vi "Periodic Tasks.vi"(8 "error in (no error)":errorcluster) -> ()   [LabVIEW 2011]
doc: "This VI runs in parallel to other tasks. It can contain as many user-defined periodic loops as you need. These can carry out PID or other sorts of timed response."
uses:
  <vilib>/addons/Kinect/SkeletonVertexTrackState.ctl
  <vilib>/Rock Robotics/SystemInterfaces/Utilities/FPGA_UtilitiesLED State.ctl
  <vilib>/Rock Robotics/SystemInterfaces/Utilities/FPGA_UtilitiesLED Source.ctl
  <vilib>/Rock Robotics/WPI/Solenoid/WPI_SolenoidValue.ctl
  <vilib>/Rock Robotics/WPI/CAN/Jaguar/SubVIs/WPI_CANJaguar_StatusSelect.ctl
  <vilib>/Rock Robotics/WPI/Compressor/WPI_CompressorGetSetRefNum.vi
  Robot Global Data.vi
  <vilib>/Rock Robotics/WPI/Solenoid/Deprecated/WPI_SolenoidGetBool.vi
  <vilib>/Rock Robotics/WPI/Solenoid/WPI_SolenoidSetEnum.vi
panel:
  out "Skeleton Tracking State":T1[](array[typedef])
  out "index":i32
  out "Target Locked":bool
  out "is not locked":bool
  out "is locked":bool
  out "Actual RPM":dbl
  out "Calculated RPM":dbl
  out "small error":bool
  out "poutput":dbl
  out "Distance from dash":dbl
  out "lr-v-out":dbl
  in  "Distance":dbl
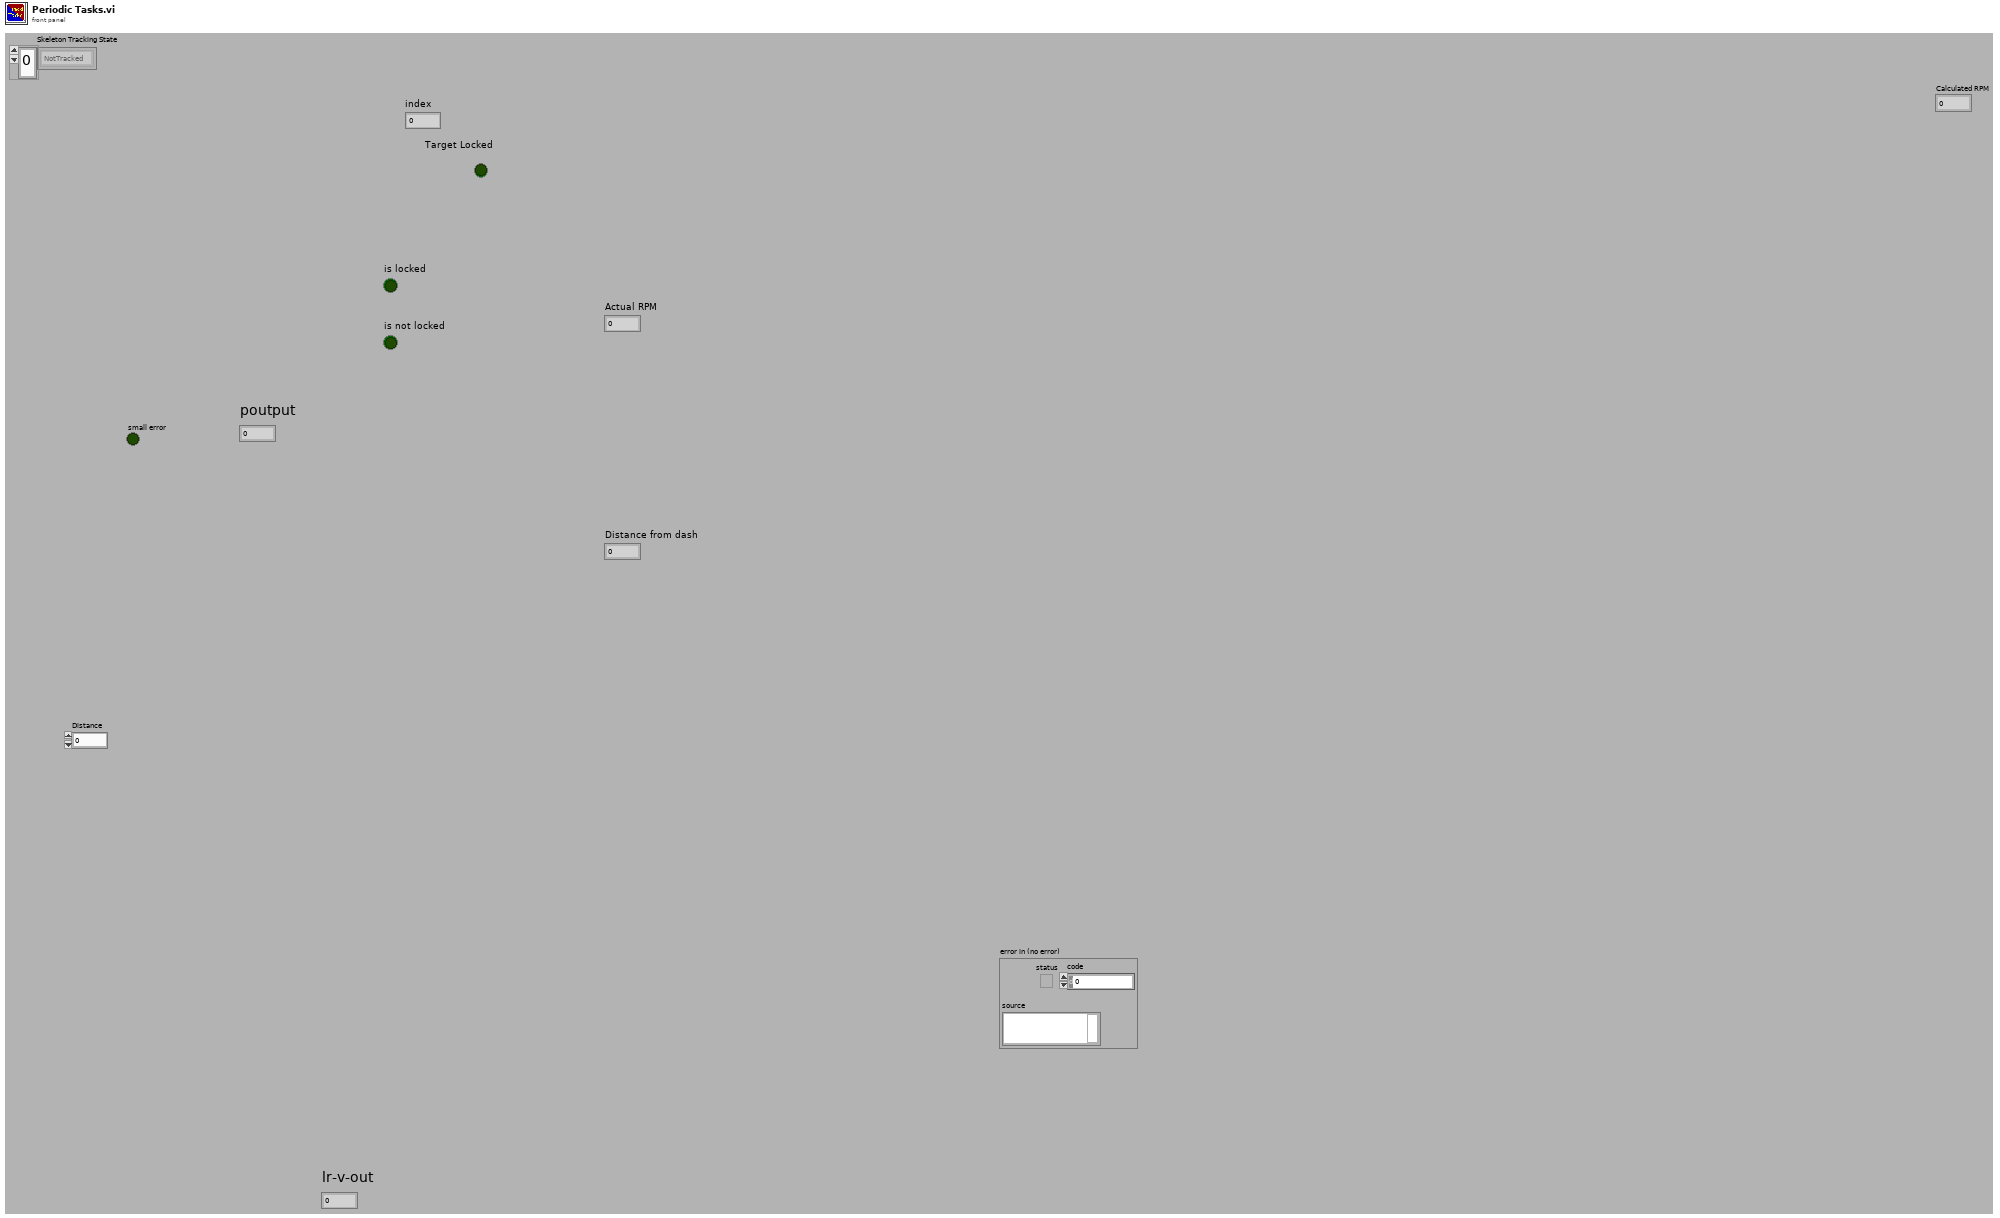
[diagram p1: front panel]
types:
  T1 = typedef "SkeletonVertexTrackState.ctl" = enum32{"NotTracked", "Inferred", "Tracked"}
  T2 = typedef "FPGA_UtilitiesLED State.ctl" = enum16{"Off", "On", "Toggle"}
  T3 = typedef "FPGA_UtilitiesLED Source.ctl" = enum16{"User LED", "FPGA LED"}
  T4 = typedef "WPI_CompressorDevRef.ctl" = cluster{"DevStatus":errorcluster, "DigitalInputDevRef":T5, "RelayDevRef":T8}
  T5 = typedef "WPI_DigitalInputDevRef.ctl" = cluster{"DevStatus":errorcluster, "DIO Channel":T6, "Digital Module":T7}
  T6 = typedef "FPGA_DIOChannel.ctl" = enum8{"DIO 1", "DIO 2", "DIO 3", "DIO 4", "DIO 5", "DIO 6", "DIO 7", "DIO 8", "DIO 9", "DIO 10", "DIO 11", "DIO 12", "DIO 13", "DIO 14", "Invalid"}
  T7 = typedef "FPGA_TypedefDigitalModule.ctl" = enum16{"Digital Module 1", "Digital Module 2"}
  T8 = typedef "WPI_RelayDevRef.ctl" = cluster{"DevStatus":errorcluster, "Relay Channel":T9, "Digital Module":T7, "Relay Direction":T10}
  T9 = typedef "FPGA_DIORelayChannel.ctl" = enum8{"Relay 1", "Relay 2", "Relay 3", "Relay 4", "Relay 5", "Relay 6", "Relay 7", "Relay 8", "Invalid"}
  T10 = typedef "WPI_RelayDirection.ctl" = enum16{"Both directions", "Forward only", "Reverse only"}
  T11 = typedef "WPI_SolenoidValue.ctl" = enum16{"Off", "On", "Forward", "Reverse"}
  T12 = typedef "WPI_JoystickDevRef.ctl" = cluster{"Device":T13}
  T13 = typedef "WPI_JoystickDeviceEnum.ctl" = enum16{"USB 1", "USB 2", "USB 3", "USB 4", "Kinect 1", "Kinect 2"}
  T14 = cluster{"axis 1 (x)":dbl, "axis 2 (y)":dbl, "axis 3 (throttle)":dbl, "axis 4":dbl, "axis 5":dbl, "axis 6":dbl}
  T15 = cluster{"RightAxis":dbl, "LeftAxis":dbl, "RightHead":bool, "Left Head":bool, "Left Leg Out":bool, "Left Leg Forward":bool, "Left Leg Back":bool, "Right Leg Out":bool, "Right Leg Forward":bool, "Right Leg Back":bool}
  T16 = typedef "WPI_SolenoidDevRef.ctl" = cluster{"DevStatus":errorcluster, "Solenoid Module":T17, "Forward Solenoid Channel":T18, "Reverse Solenoid Channel":T18}
  T17 = typedef "FPGA_TypedefSolenoidModule.ctl" = enum16{"Solenoid Module 1", "Solenoid Module 2"}
  T18 = typedef "WPI_SolenoidChannel.ctl" = enum8{"Solenoid 1", "Solenoid 2", "Solenoid 3", "Solenoid 4", "Solenoid 5", "Solenoid 6", "Solenoid 7", "Solenoid 8", "Invalid"}
  T19 = typedef "WPI_JoystickButtonState.ctl" = cluster{"Button 1":bool, "Button 2":bool, "Button 3":bool, "Button 4":bool, "Button 5":bool, "Button 6":bool, "Button 7":bool, "Button 8":bool, "Button 9":bool, "Button 10":bool, "Button 11":bool, "Button 12":bool}
  T20 = typedef "WPI_CANJaguar_StatusSelect.ctl" = enum16{"Output Percent VBus", "Output Voltage", "Bus Voltage", "Current", "Temperature", "Position", "Speed", "Limit Switches", "Faults", "Fault Counters", "Power Cycle"}
  T21 = typedef "WPI_MotorControlDeviceRef.ctl" = cluster{"DeviceStatus":errorcluster, "Type":enum16{"PWM", "CAN"}, "PWM":cluster{"Digital Module":T7, "PWM Channel":T22, "DeadBand":T23}, "CAN":cluster{"Device Number":u8, "Control Mode":T24, "Semaphore":T25, "Max Vout":dbl}, "Invert":bool, "TransformRef":T26, "InvTransformRef":T26}
  T22 = typedef "FPGA_DIOPWMChannel.ctl" = enum8{"PWM 1", "PWM 2", "PWM 3", "PWM 4", "PWM 5", "PWM 6", "PWM 7", "PWM 8", "PWM 9", "PWM 10", "Invalid"}
  T23 = typedef "WPI_PWMDeadband.ctl" = cluster{"Name":string, "maxPositivePwm":i32, "minPositivePwm":i32, "centerPwm":i32, "maxNegativePwm":i32, "minNegativePwm":i32, "angularRange":u16}
  T24 = typedef "WPI_CANJaguar_ControlMode.ctl" = enum8{"Percent VBus", "Current", "Speed", "Position", "Voltage"}
  T25 = typedef "Semaphore RefNum" = refnum<k1>
  T26 = typedef "WPI_PWMTransform_ConPane.ctl" = refnum<vi>
  T27 = typedef "WPI_CANJaguar_Status.ctl" = cluster{"Output Percent VBus":dbl, "Output Voltage":dbl, "Bus Voltage":dbl, "Current":dbl, "Temperature":dbl, "Position":dbl, "Speed":dbl, "Limits":cluster{"Forward Limit":bool, "Reverse Limit":bool, "Forward Soft Limit":bool, "Reverse Soft Limit":bool, "Sticky Forward Limit":bool, "Sticky Reverse Limit":bool, "Sticky Forward Soft Limit":bool, "Sticky Reverse Soft Limit":bool}, "Faults":cluster{"Current Fault":bool, "Temperature Fault":bool, "Bus Voltage Fault":bool, "Gate Driver Fault":bool, "Comm Fault":bool}, "Fault Counters":cluster{"Current Faults":u8, "Temperature Faults":u8, "Bus Voltage Faults":u8, "Gate Driver Faults":u8, "Comm Faults":u8, "CAN Status":u8, "CAN RX Errors":u8, "CAN TX Errors":u8}, "Power Cycle":bool}
  T28 = typedef "WPI_DigitalOutputDevRef.ctl" = cluster{"Digital Module":T7, "DIO Channel":T6, "DevStatus":errorcluster}
  T29 = cluster{"Selected Distance":dbl, "Calculated RPM":dbl, "Actual RPM":dbl, "Target Locked":bool}
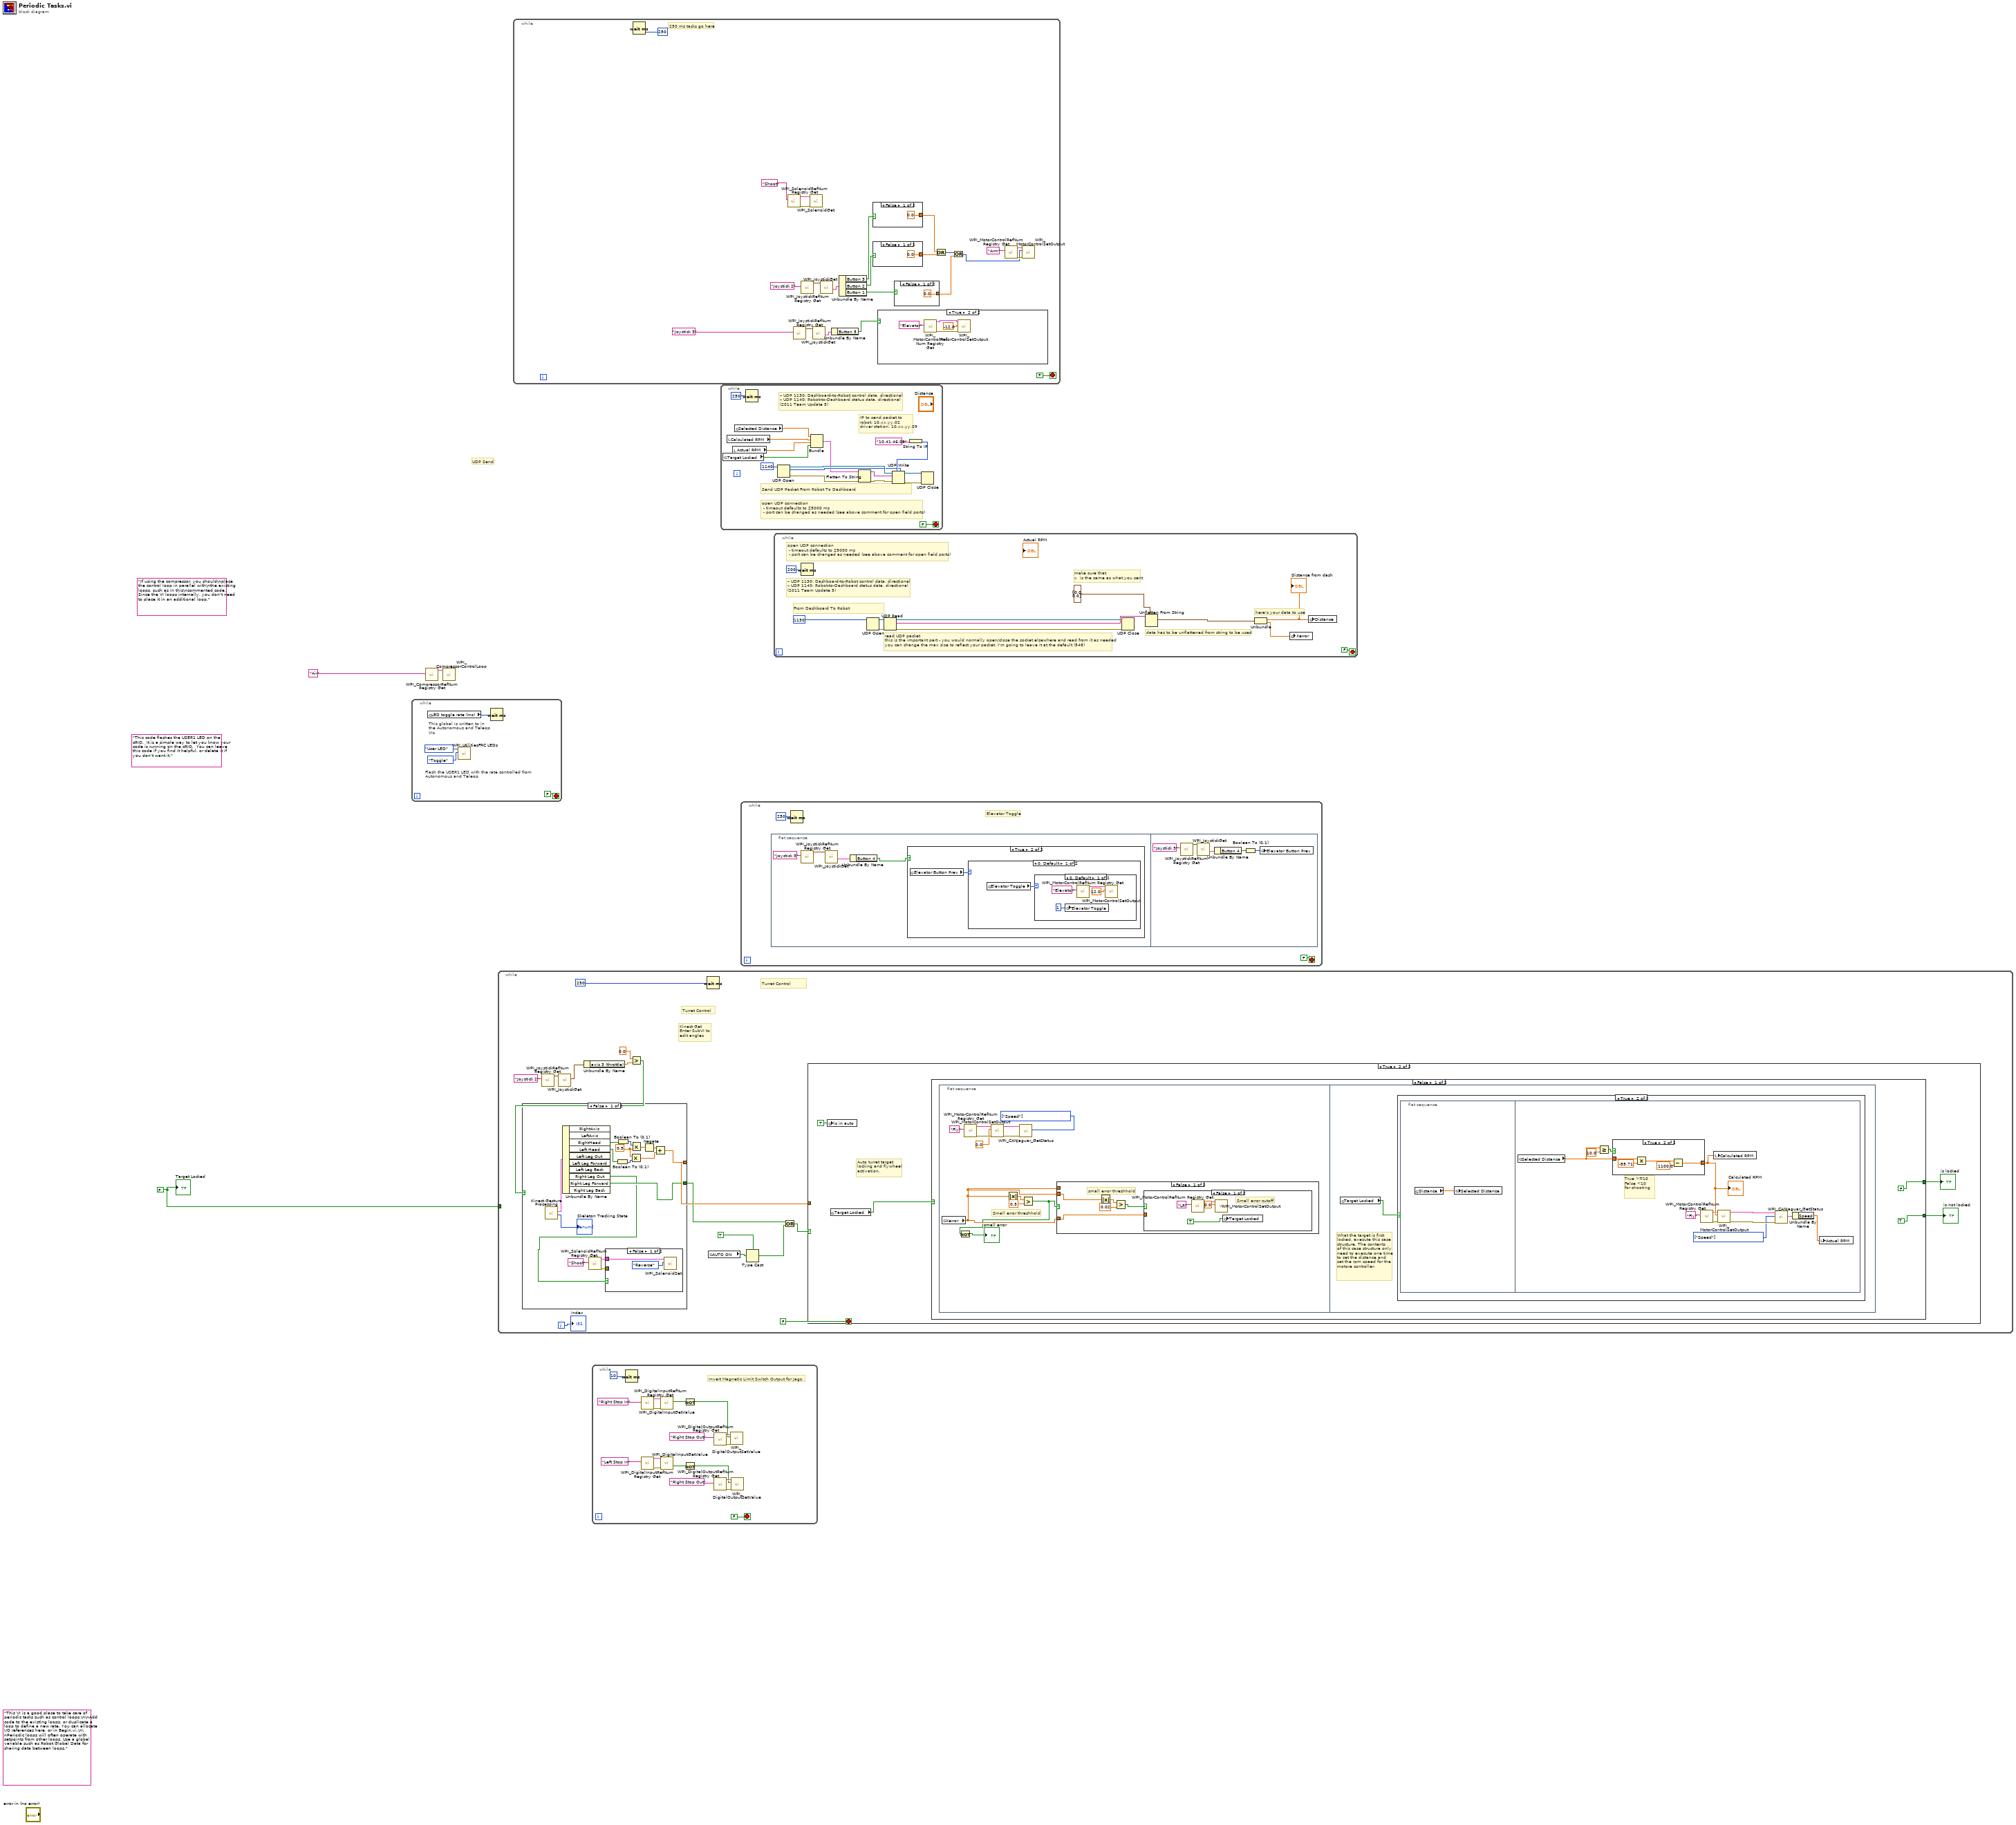
[diagram p0: block diagram]
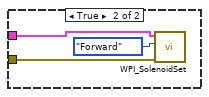
[diagram p2: hidden frame]
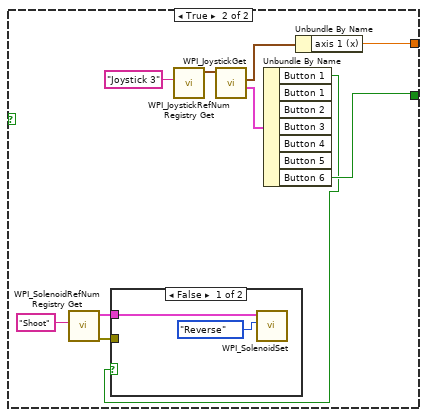
[diagram p3: hidden frame]
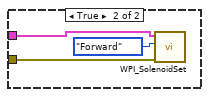
[diagram p4: hidden frame]
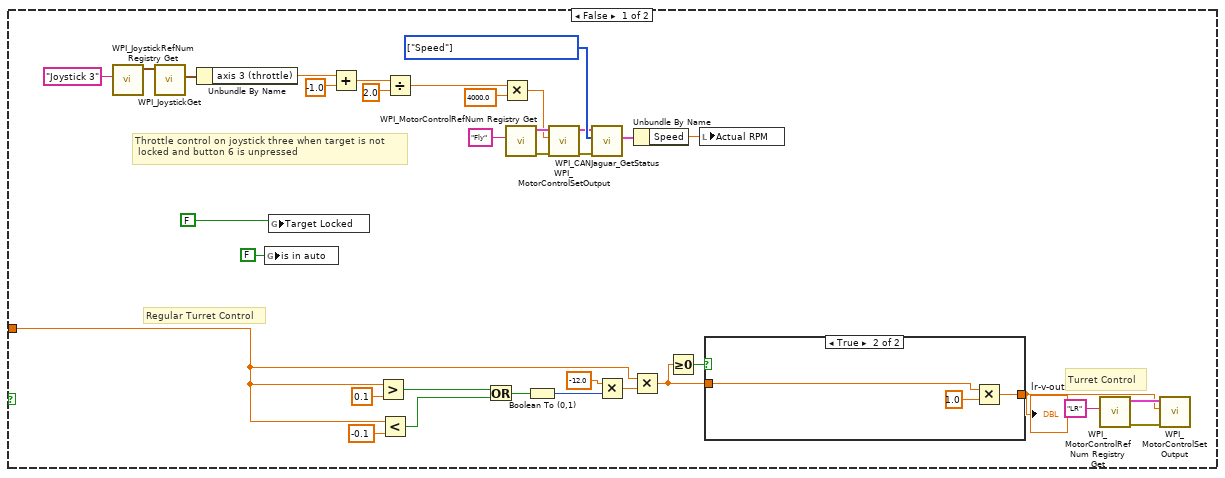
[diagram p5: hidden frame]
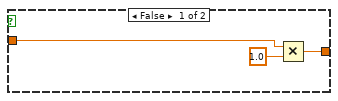
[diagram p6: hidden frame]
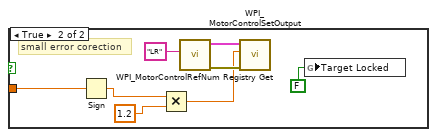
[diagram p7: hidden frame]
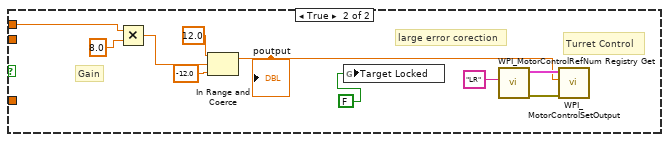
[diagram p8: hidden frame]
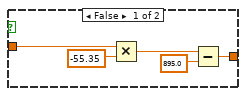
[diagram p10: hidden frame]
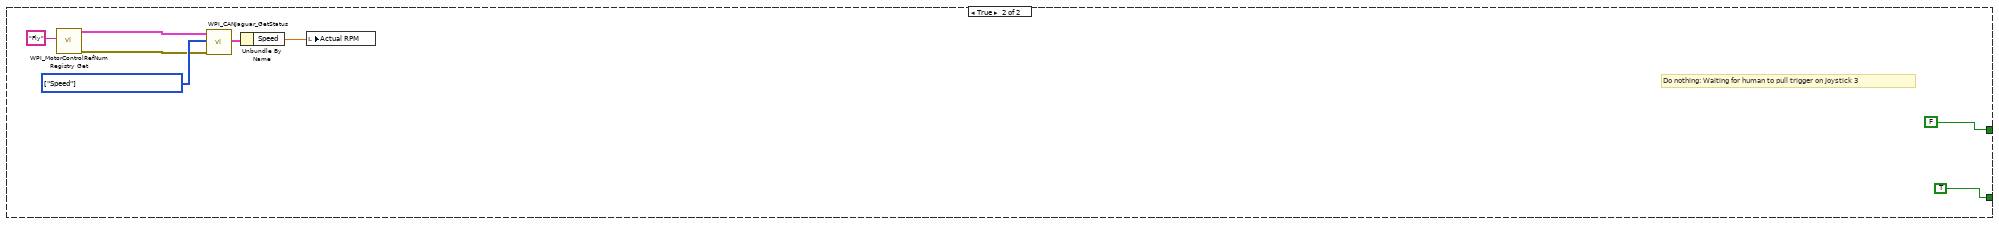
[diagram p11: hidden frame]
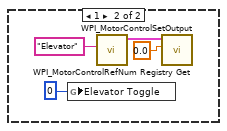
[diagram p13: hidden frame]
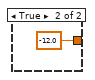
[diagram p15: hidden frame]
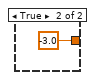
[diagram p16: hidden frame]
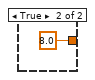
[diagram p17: hidden frame]
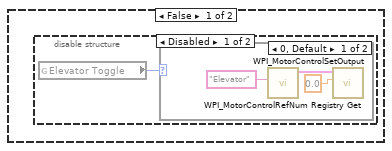
[diagram p18: hidden frame]
diagram:
  w3 = FALSE ("Target Locked")
  (unwired) "This VI is a good place to take care of periodic tasks such as control loops.\n\nAdd code to the existing loops, or duplicate a loop to define a new rate. You can allocate I/O references here, or in Begin.vi.\n\nPeriodic loops will often operate with setpoints from other loops. Use a global variable such as Robot Global Data for sharing data between loops."
  (unwired) "If using the compressor, you should\nplace the control loop in parallel with\nthe existing loops, such as in this\ncommented code. Since the VI loops internally, you don't need to place it in an additional loop."
  (unwired) "This code flashes the USER1 LED on the cRIO.  It is a simple way to let you know your code is running on the cRIO.  You can leave this code if you find it helpful, or delete it if you don't want it."
  # "UDP Send"
  n1 = while {
    stop <- FALSE stop-if-true
    # "This global is written to in the Autonomous and Teleop VIs"
    # "Flash the USER1 LED with the rate controlled from Autonomous and Teleop"
    n2 = global read "Robot Global Data.vi" "LED toggle rate (ms)"() -> (w4:u32)
    n3 = call <vilib>:"WPI_UtilitiesFRC LEDs.vi"("State"=FPGA_UtilitiesLED_State."Toggle", "LED Type"=FPGA_UtilitiesLED_Source."User LED") -> ()  [unwired: 1 in, 9 out]
    n4 = Wait (ms)(milliseconds to wait=w4) -> ()  [unwired: 1 out]
  }
  n5 = call <vilib>:"WPI_CompressorRefNum Registry Get.vi"("refnum name"="Air") -> ("CompressorDevRef"=w2:T4)  [unwired: 9 in, 1 out]
  n6 = call <vilib>:"WPI_CompressorControlLoop.vi"("CompressorDevRef"=w2) -> ()  [unwired: 11 in]
  n7 = while {
    tunnel: w3 -> [_]
    i -> [w20]
    stop <- FALSE stop-if-true
    # "Kinect Get\nEnter SubVI to edit angles"
    # "Turret Control"
    # "Turret Control"
    n8 = call <vilib>:"WPI_JoystickRefNum Registry Get.vi"("refnum name"="Joystick 2") -> ("JoystickDevRef"=w12:T12)  [unwired: 9 in, 1 out]
    n9 = call <vilib>:"WPI_JoystickGet.vi"("JoystickDevRef"=w12) -> ("Axes"=w11:T14)  [unwired: 4 in, 2 out]
    n10 = Unbundle By Name(w11) -> ("axis 3 (throttle)"=w9:dbl)
    n11 = Greater?(x=0.0, y=w9) -> (0:w8:bool)
    n12 = case shown="False" w8 {
      tunnel: [w31 w50] -> w15
      tunnel: [w32 w48] -> w14
      frame False {
        w33 = 0.5 ("y")
        n13 = call "Kinect Gesture Processing.vi"() -> ("Skeleton Tracking State"=→"Skeleton Tracking State":T1[], "Joystick Data"=w38:T15)  [unwired: 7 in, 1 out]
        n14 = Unbundle By Name(w38) -> ("RightHead"=w37:bool, "Left Head"=w36:bool, "Right Leg Out"=w23:bool, "Right Leg Forward"=w31:bool)  [unwired: 6 out]
        n15 = call <vilib>:"WPI_SolenoidRefNum Registry Get.vi"("refnum name"="Shoot") -> ("error out"=w24:errorcluster, "SolenoidDevRef"=w25:T16)  [unwired: 9 in]
        n16 = case shown="False" w23 {
          tunnel: w25 -> [w39 w42]
          tunnel: w24 -> [_ w41]
          frame False {
            n17 = call-poly <vilib>:"WPI_SolenoidSet.vi"("Value"=WPI_SolenoidValue."Reverse", "SolenoidDevRef"=w39) -> ()  [unwired: 8 in, 2 out]
          }
          frame True {
            n18 = call-poly <vilib>:"WPI_SolenoidSet.vi"("error in (no error)"=w41, "Value"=WPI_SolenoidValue."Forward", "SolenoidDevRef"=w42) -> ()  [unwired: 7 in, 2 out]
          }
        }
        n19 = Boolean To (0,1)(Boolean=w36) -> (0, 1=w34:i16)
        n20 = Boolean To (0,1)(Boolean=w37) -> (0, 1=w35:i16)
        n21 = Multiply(x=w33, y=w34) -> (x*y=w27:dbl)
        n22 = Multiply(x=w35, y=w33) -> (x*y=w29:dbl)
        n23 = Negate(x=w29) -> (-x=w28:dbl)
        n24 = Add(x=w28, y=w27) -> (x+y=w32:dbl)
      }
      frame True {
        n25 = call <vilib>:"WPI_SolenoidRefNum Registry Get.vi"("refnum name"="Shoot") -> ("error out"=w45:errorcluster, "SolenoidDevRef"=w46:T16)  [unwired: 9 in]
        n26 = call <vilib>:"WPI_JoystickRefNum Registry Get.vi"("refnum name"="Joystick 3") -> ("JoystickDevRef"=w51:T12)  [unwired: 9 in, 1 out]
        n27 = call <vilib>:"WPI_JoystickGet.vi"("JoystickDevRef"=w51) -> ("Buttons"=w53:T19, "Axes"=w49:T14)  [unwired: 4 in, 1 out]
        n28 = Unbundle By Name(w53) -> ("Button 1"=w44:bool, "Button 6"=w50:bool)  [unwired: 5 out]
        n29 = case shown="False" w44 {
          tunnel: w46 -> [w54 w57]
          tunnel: w45 -> [_ w56]
          frame False {
            n30 = call-poly <vilib>:"WPI_SolenoidSet.vi"("Value"=WPI_SolenoidValue."Reverse", "SolenoidDevRef"=w54) -> ()  [unwired: 8 in, 2 out]
          }
          frame True {
            n31 = call-poly <vilib>:"WPI_SolenoidSet.vi"("error in (no error)"=w56, "Value"=WPI_SolenoidValue."Forward", "SolenoidDevRef"=w57) -> ()  [unwired: 7 in, 2 out]
          }
        }
        n32 = Unbundle By Name(w49) -> ("axis 1 (x)"=w48:dbl)
      }
    }
    n33 = Wait (ms)(milliseconds to wait=u32 250) -> ()  [unwired: 1 out]
    n34 = global read "Robot Global Data.vi" "AUTO ON"() -> (w18:bool)
    n35 = Type Cast(type=TRUE, x=w18) -> (*(type *) &x=w16:bool)
    n36 = Or(x=w15, y=w16) -> (x .or. y?=w19:bool)
    n37 = case shown="True" w19 {
      tunnel: w14 -> [w59 _]
      frame False {
        w74 = T20[] [enum."Speed"] items=["Output Percent VBus", "Output Voltage", "Bus Voltage", "Current", "Temperature", "Position", "Speed", "Limit Switches", "Faults", "Fault Counters", "Power Cycle"] ("Status Select")
        # "Throttle control on joystick three when target is not\n locked and button 6 is unpressed"
        # "Regular Turret Control"
        # "Turret Control"
        n38 = call <vilib>:"WPI_JoystickRefNum Registry Get.vi"("refnum name"="Joystick 3") -> ("JoystickDevRef"=w70:T12)  [unwired: 9 in, 1 out]
        n39 = call <vilib>:"WPI_JoystickGet.vi"("JoystickDevRef"=w70) -> ("Axes"=w71:T14)  [unwired: 4 in, 2 out]
        n40 = Unbundle By Name(w71) -> ("axis 3 (throttle)"=w68:dbl)
        n41 = global write "Robot Global Data.vi" "is in auto"(FALSE ("is in auto")) -> ()
        n42 = global write "Robot Global Data.vi" "Target Locked"(FALSE ("Target Locked")) -> ()
        n43 = Add(x=w68, y=-1.0) -> (x+y=w66:dbl)
        n44 = Greater?(x=w59, y=0.1) -> (0:w87:bool)
        n45 = Less?(x=w59, y=-0.1) -> (x < y?=w86:bool)
        n46 = Divide(x=w66, y=2.0) -> (x/y=w60:dbl)
        n47 = Or(x=w87, y=w86) -> (x .or. y?=w85:bool)
        n48 = Multiply(x=w60, y=4000.0) -> (x*y=w63:dbl)
        n49 = call <vilib>:"WPI_MotorControlRefNum Registry Get.vi"("refnum name"="Fly") -> ("error out"=w75:errorcluster, "MotorControlDevRef"=w76:T21)  [unwired: 9 in]
        n50 = Boolean To (0,1)(Boolean=w85) -> (0, 1=w84:i16)
        n51 = call <vilib>:"WPI_MotorControlSetOutput.vi"("error in (no error)"=w75, "Output"=w63, "MotorControlDevRef"=w76) -> ("error out"=w72:errorcluster, "MotorControlDevRef"=w73:T21)  [unwired: 7 in]
        n52 = call <vilib>:"WPI_CANJaguar_GetStatus.vi"("error in (no error)"=w72, "Status Select"=w74, "CAN Jaguar Ref"=w73) -> ("Status"=w62:T27)  [unwired: 6 in, 2 out]
        n53 = Multiply(x=-12.0, y=w84) -> (x*y=w83:dbl)
        n54 = Multiply(x=w59, y=w83) -> (x*y=w81:dbl)
        n55 = Unbundle By Name(w62) -> ("Speed"=w61:dbl)
        n56 = Greater Or Equal To 0?(x=w81) -> (x >= 0?=w82:bool)
        n57 = local write "Actual RPM"(w61) -> ()
        n58 = case shown="True" w82 {
          tunnel: w81 -> [w96 w99]
          tunnel: [w95 w98] -> w80
          frame False {
            n59 = Multiply(x=w96, y=1.0) -> (x*y=w95:dbl)
          }
          frame True {
            n60 = Multiply(x=w99, y=1.0) -> (x*y=w98:dbl)
          }
        }
        "lr-v-out" <- w80
        n61 = call <vilib>:"WPI_MotorControlRefNum Registry Get.vi"("refnum name"="LR") -> ("error out"=w92:errorcluster, "MotorControlDevRef"=w93:T21)  [unwired: 9 in]
        n62 = call <vilib>:"WPI_MotorControlSetOutput.vi"("error in (no error)"=w92, "Output"=w80, "MotorControlDevRef"=w93) -> ()  [unwired: 7 in, 2 out]
      }
      frame True {
        # "Auto turret target\nlocking and flywheel\nactivation."
        n63 = global write "Robot Global Data.vi" "is in auto"(TRUE ("is in auto")) -> ()
        n64 = global read "Robot Global Data.vi" "Target Locked"() -> (w100:bool)
        n65 = case shown="False" w100 {
          tunnel: [FALSE FALSE] -> w102
          tunnel: [TRUE TRUE] -> w101
          frame False {
            n66 = flat-sequence {
              frame #0 {
                w114 = T20[] [enum."Speed"] items=["Output Percent VBus", "Output Voltage", "Bus Voltage", "Current", "Temperature", "Position", "Speed", "Limit Switches", "Faults", "Fault Counters", "Power Cycle"] ("Status Select")
                # "Small error threshhold"
                n67 = global read "Robot Global Data.vi" "Xerror"() -> (w110:dbl)
                n68 = call <vilib>:"WPI_MotorControlRefNum Registry Get.vi"("refnum name"="Fly") -> ("error out"=w115:errorcluster, "MotorControlDevRef"=w116:T21)  [unwired: 9 in]
                n69 = call <vilib>:"WPI_MotorControlSetOutput.vi"("error in (no error)"=w115, "Output"=0.0, "MotorControlDevRef"=w116) -> ("error out"=w111:errorcluster, "MotorControlDevRef"=w112:T21)  [unwired: 7 in]
                n70 = Absolute Value(x=w110) -> (abs(x)=w106:dbl)
                n71 = call <vilib>:"WPI_CANJaguar_GetStatus.vi"("error in (no error)"=w111, "Status Select"=w114, "CAN Jaguar Ref"=w112) -> ()  [unwired: 6 in, 3 out]
                n72 = Greater?(x=w106, y=0.3) -> (0:w109:bool)
                n73 = Not(x=w109) -> (.not. x?=→"small error":bool)
                n74 = case shown="False" w109 {
                  tunnel: w110 -> [_ w140]
                  tunnel: w110 -> [w122 _]
                  tunnel: w110 -> [w119 _]
                  frame False {
                    # "small error threshhold"
                    n75 = Absolute Value(x=w119) -> (abs(x)=w121:dbl)
                    n76 = Greater?(x=w121, y=0.02) -> (0:w118:bool)
                    n77 = case shown="False" w118 {
                      tunnel: w122 -> [_ w131]
                      frame False {
                        # "Small error cutoff"
                        n78 = call <vilib>:"WPI_MotorControlRefNum Registry Get.vi"("refnum name"="LR") -> ("MotorControlDevRef"=w126:T21)  [unwired: 9 in, 1 out]
                        n79 = call <vilib>:"WPI_MotorControlSetOutput.vi"("Output"=0.0, "MotorControlDevRef"=w126) -> ()  [unwired: 8 in, 2 out]
                        n80 = global write "Robot Global Data.vi" "Target Locked"(TRUE ("Target Locked")) -> ()
                      }
                      frame True {
                        # "small error corection"
                        n81 = Sign(1:w131) -> (0:w130:dbl)
                        n82 = Multiply(x=w130, y=1.2) -> (x*y=w129:dbl)
                        n83 = call <vilib>:"WPI_MotorControlRefNum Registry Get.vi"("refnum name"="LR") -> ("error out"=w133:errorcluster, "MotorControlDevRef"=w134:T21)  [unwired: 9 in]
                        n84 = call <vilib>:"WPI_MotorControlSetOutput.vi"("error in (no error)"=w133, "Output"=w129, "MotorControlDevRef"=w134) -> ()  [unwired: 7 in, 2 out]
                        n85 = global write "Robot Global Data.vi" "Target Locked"(FALSE ("Target Locked")) -> ()
                      }
                    }
                  }
                  frame True {
                    # "large error corection"
                    # "Gain"
                    # "Turret Control"
                    n86 = Multiply(x=w140, y=8.0) -> (x*y=w137:dbl)
                    n87 = In Range and Coerce(upper limit=12.0, x=w137, lower limit=-12.0) -> (coerced(x)=w139:dbl)  [unwired: 1 out]
                    "poutput" <- w139
                    n88 = global write "Robot Global Data.vi" "Target Locked"(FALSE ("Target Locked")) -> ()
                    n89 = call <vilib>:"WPI_MotorControlRefNum Registry Get.vi"("refnum name"="LR") -> ("error out"=w143:errorcluster, "MotorControlDevRef"=w144:T21)  [unwired: 9 in]
                    n90 = call <vilib>:"WPI_MotorControlSetOutput.vi"("error in (no error)"=w143, "Output"=w139, "MotorControlDevRef"=w144) -> ()  [unwired: 7 in, 2 out]
                  }
                }
              }
              frame #1 {
                # "What the target is first\nlocked, execute this case\nstructure. The contents\nof this case structure only\nneed to execute one time\nto set the distance and\nset the rpm speed for the\nmotore controller."
                n91 = global read "Robot Global Data.vi" "Target Locked"() -> (w145:bool)
                n92 = case shown="True" w145 {
                  frame False {
                  }
                  frame True {
                    n93 = flat-sequence {
                      frame #0 {
                        n94 = global read "Robot Global Data.vi" "Distance"() -> (w146:dbl)
                        n95 = global write "Robot Global Data.vi" "Selected Distance"(w146) -> ()
                      }
                      frame #1 {
                        w151 = T20[] [enum."Speed"] items=["Output Percent VBus", "Output Voltage", "Bus Voltage", "Current", "Temperature", "Position", "Speed", "Limit Switches", "Faults", "Fault Counters", "Power Cycle"] ("Status Select")
                        # "True >=10\nFalse <10\nfor shooting"
                        n96 = global read "Robot Global Data.vi" "Selected Distance"() -> (w149:dbl)
                        n97 = Greater Or Equal?(x=w149, y=10.0) -> (x >= y?=w154:bool)
                        n98 = case shown="True" w154 {
                          tunnel: w149 -> [w159 w164]
                          tunnel: [w163 w168] -> w148
                          frame False {
                            n99 = Multiply(x=w159, y=-55.35) -> (x*y=w161:dbl)
                            n100 = Subtract(x=w161, y=895.0) -> (x-y=w163:dbl)
                          }
                          frame True {
                            n101 = Multiply(x=w164, y=-55.71) -> (x*y=w166:dbl)
                            n102 = Subtract(x=w166, y=1100.0) -> (x-y=w168:dbl)
                          }
                        }
                        "Calculated RPM" <- w148
                        n103 = call <vilib>:"WPI_MotorControlRefNum Registry Get.vi"("refnum name"="Fly") -> ("error out"=w156:errorcluster, "MotorControlDevRef"=w157:T21)  [unwired: 9 in]
                        n104 = local write "Calculated RPM"(w148) -> ()
                        n105 = call <vilib>:"WPI_MotorControlSetOutput.vi"("error in (no error)"=w156, "Output"=w148, "MotorControlDevRef"=w157) -> ("error out"=w152:errorcluster, "MotorControlDevRef"=w153:T21)  [unwired: 7 in]
                        n106 = call <vilib>:"WPI_CANJaguar_GetStatus.vi"("error in (no error)"=w152, "Status Select"=w151, "CAN Jaguar Ref"=w153) -> ("Status"=w150:T27)  [unwired: 6 in, 2 out]
                        n107 = Unbundle By Name(w150) -> ("Speed"=w147:dbl)
                        n108 = local write "Actual RPM"(w147) -> ()
                      }
                    }
                  }
                }
              }
            }
          }
          frame True {
            w175 = T20[] [enum."Speed"] items=["Output Percent VBus", "Output Voltage", "Bus Voltage", "Current", "Temperature", "Position", "Speed", "Limit Switches", "Faults", "Fault Counters", "Power Cycle"] ("Status Select")
            # "Do nothing: Waiting for human to pull trigger on Joystick 3"
            n109 = call <vilib>:"WPI_MotorControlRefNum Registry Get.vi"("refnum name"="Fly") -> ("error out"=w171:errorcluster, "MotorControlDevRef"=w172:T21)  [unwired: 9 in]
            n110 = call <vilib>:"WPI_CANJaguar_GetStatus.vi"("error in (no error)"=w171, "Status Select"=w175, "CAN Jaguar Ref"=w172) -> ("Status"=w174:T27)  [unwired: 6 in, 2 out]
            n111 = Unbundle By Name(w174) -> ("Speed"=w173:dbl)
            n112 = local write "Actual RPM"(w173) -> ()
          }
        }
        "is locked" <- w102
        "is not locked" <- w101
      }
    }
    "index" <- w20
  }
  n113 = while {
    stop <- FALSE stop-if-true
    # "250 ms tasks go here"
    n114 = Wait (ms)(milliseconds to wait=u32 250) -> ()  [unwired: 1 out]
    n115 = call <vilib>:"WPI_SolenoidRefNum Registry Get.vi"("refnum name"="Shoot") -> ("error out"=w194:errorcluster, "SolenoidDevRef"=w196:T16)  [unwired: 9 in]
    n116 = call <vilib>:"WPI_JoystickRefNum Registry Get.vi"("refnum name"="Joystick 3") -> ("JoystickDevRef"=w178:T12)  [unwired: 9 in, 1 out]
    n117 = call <vilib>:"WPI_JoystickRefNum Registry Get.vi"("refnum name"="Joystick 2") -> ("JoystickDevRef"=w192:T12)  [unwired: 9 in, 1 out]
    n118 = call-poly <vilib>:"WPI_SolenoidGet.vi"("error in (no error)"=w194, "SolenoidDevRef"=w196) -> ()  [unwired: 7 in, 3 out]
    n119 = call <vilib>:"WPI_JoystickGet.vi"("JoystickDevRef"=w178) -> ("Buttons"=w180:T19)  [unwired: 4 in, 2 out]
    n120 = call <vilib>:"WPI_JoystickGet.vi"("JoystickDevRef"=w192) -> ("Buttons"=w195:T19)  [unwired: 4 in, 2 out]
    n121 = Unbundle By Name(w180) -> ("Button 5"=w177:bool)
    n122 = Unbundle By Name(w195) -> ("Button 3"=w188:bool, "Button 2"=w187:bool, "Button 1"=w186:bool)
    n123 = case shown="False" w188 {
      tunnel: [0.0 ("Output") 8.0 ("Output")] -> w184
      frame False {
      }
      frame True {
      }
    }
    n124 = case shown="False" w187 {
      tunnel: [0.0 ("Output") -3.0 ("Output")] -> w185
      frame False {
      }
      frame True {
      }
    }
    n125 = case shown="True" w177 {
      frame False {
        n126 = disable-structure shown="Disabled" {
          frame Disabled {
            n127 = global read "Robot Global Data.vi" "Elevator Toggle"() -> (w206:u8)
            n128 = case shown="0, Default" w206 {
              frame 0, Default {
                n129 = call <vilib>:"WPI_MotorControlRefNum Registry Get.vi"("refnum name"="Elevator") -> ("MotorControlDevRef"=w208:T21)  [unwired: 9 in, 1 out]
                n130 = call <vilib>:"WPI_MotorControlSetOutput.vi"("Output"=0.0 ("y"), "MotorControlDevRef"=w208) -> ()  [unwired: 8 in, 2 out]
              }
              frame 1 {
              }
            }
          }
          frame Enabled {
          }
        }
      }
      frame True {
        n131 = call <vilib>:"WPI_MotorControlRefNum Registry Get.vi"("refnum name"="Elevator") -> ("error out"=w210:errorcluster, "MotorControlDevRef"=w212:T21)  [unwired: 9 in]
        n132 = call <vilib>:"WPI_MotorControlSetOutput.vi"("error in (no error)"=w210, "Output"=-12.0 ("y"), "MotorControlDevRef"=w212) -> ()  [unwired: 7 in, 2 out]
      }
    }
    n133 = case shown="False" w186 {
      tunnel: [0.0 ("Output") -12.0 ("Output")] -> w183
      frame False {
      }
      frame True {
      }
    }
    n134 = Or(x=w184, y=w185) -> (x .or. y?=w182:i32)
    n135 = Or(x=w182, y=w183) -> (x .or. y?=w181:i32)
    n136 = call <vilib>:"WPI_MotorControlRefNum Registry Get.vi"("refnum name"="Arm") -> ("error out"=w190:errorcluster, "MotorControlDevRef"=w191:T21)  [unwired: 9 in]
    n137 = call <vilib>:"WPI_MotorControlSetOutput.vi"("error in (no error)"=w190, "Output"=w181, "MotorControlDevRef"=w191) -> ()  [unwired: 7 in, 2 out]
  }
  n138 = while {
    stop <- FALSE stop-if-true
    # "Invert Magnetic Limit Switch Output for Jags."
    n139 = Wait (ms)(milliseconds to wait=u32 10) -> ()  [unwired: 1 out]
    n140 = call <vilib>:"WPI_DigitalInputRefNum Registry Get.vi"("refnum name"="Right Stop In") -> ("error out"=w224:errorcluster, "DigitalInputDevRef"=w227:T5)  [unwired: 9 in]
    n141 = call <vilib>:"WPI_DigitalInputRefNum Registry Get.vi"("refnum name"="Left Stop In") -> ("error out"=w225:errorcluster, "DigitalInputDevRef"=w228:T5)  [unwired: 9 in]
    n142 = call <vilib>:"WPI_DigitalInputGetValue.vi"("error in (no error)"=w224, "DigitalInputDevRef"=w227) -> ("Value"=w215:bool)  [unwired: 7 in, 2 out]
    n143 = call <vilib>:"WPI_DigitalInputGetValue.vi"("error in (no error)"=w225, "DigitalInputDevRef"=w228) -> ("Value"=w217:bool)  [unwired: 7 in, 2 out]
    n144 = Not(x=w215) -> (.not. x?=w214:bool)
    n145 = Not(x=w217) -> (.not. x?=w216:bool)
    n146 = call <vilib>:"WPI_DigitalOutputRefNum Registry Get.vi"("refnum name"="Right Stop Out") -> ("error out"=w219:errorcluster, "DigitalOutputDevRef"=w218:T28)  [unwired: 9 in]
    n147 = call <vilib>:"WPI_DigitalOutputRefNum Registry Get.vi"("refnum name"="Right Stop Out") -> ("error out"=w221:errorcluster, "DigitalOutputDevRef"=w220:T28)  [unwired: 9 in]
    n148 = call <vilib>:"WPI_DigitalOutputSetValue.vi"("error in (no error)"=w219, "Value"=w214, "DigitalOutputDevRef"=w218) -> ()  [unwired: 7 in, 2 out]
    n149 = call <vilib>:"WPI_DigitalOutputSetValue.vi"("error in (no error)"=w221, "Value"=w216, "DigitalOutputDevRef"=w220) -> ()  [unwired: 7 in, 2 out]
  }
  n150 = while {
    stop <- FALSE stop-if-true
    # "IP to send packet to \nrobot: 10.xx.yy.02\ndriver station: 10.xx.yy.09"
    # "open UDP connection\n - timeout defaults to 25000 ms\n - port can be changed as needed (see above comment for open field ports)"
    # "Send UDP Packet From Robot To Dashboard"
    # "– UDP 1130: Dashboard-to-Robot control data, directional\n– UDP 1140: Robot-to-Dashboard status data, directional\n(2011 Team Update 5)"
    n151 = global read "Robot Global Data.vi" "Target Locked"() -> (w232:bool)
    n152 = local read "Calculated RPM"() -> (w236:dbl)
    n153 = local read "Actual RPM"() -> (w235:dbl)
    n154 = global read "Robot Global Data.vi" "Selected Distance"() -> (w237:dbl)
    n155 = Wait (ms)(milliseconds to wait=u32 250) -> ()  [unwired: 1 out]
    n156 = UDP Open(11:u16 1140 ("port")) -> (port=w241:refnum<k16>, 0:w239:errorcluster, 2:w240:u16)  [unwired: 1 in, 3 out]
    n157 = Bundle("Selected Distance"=w237, "Calculated RPM"=w236, "Actual RPM"=w235, "Target Locked"=w232) -> (w234:T29)  [unwired: 1 in]
    n158 = Flatten To String(anything=w234, error in (no error)=w239) -> (data string=w245:string, error out=w246:errorcluster)  [unwired: 3 out]
    n159 = String To IP(1:"10.41.46.09") -> (0:w247:u32)
    n160 = UDP Write(address=w247, port or service name=w240, connection ID=w241, data in=w245, 8:w246) -> (error out=w243:errorcluster, 3:w244:refnum<k16>)  [unwired: 1 out]
    n161 = UDP Close(connection ID=w244, 8:w243) -> ()  [unwired: 2 out]
  }
  n162 = while {
    stop <- FALSE stop-if-true
    # "Elevator Toggle"
    n163 = flat-sequence {
      frame #0 {
        n164 = call <vilib>:"WPI_JoystickRefNum Registry Get.vi"("refnum name"="Joystick 3") -> ("JoystickDevRef"=w253:T12)  [unwired: 9 in, 1 out]
        n165 = call <vilib>:"WPI_JoystickGet.vi"("JoystickDevRef"=w253) -> ("Buttons"=w252:T19)  [unwired: 4 in, 2 out]
        n166 = Unbundle By Name(w252) -> ("Button 4"=w251:bool)
        n167 = case shown="True" w251 {
          frame False {
          }
          frame True {
            n168 = global read "Robot Global Data.vi" "Elevator Button Prev"() -> (w255:u8)
            n169 = case shown="0, Default" w255 {
              frame 0, Default {
                n170 = global read "Robot Global Data.vi" "Elevator Toggle"() -> (w256:u8)
                n171 = case shown="0, Default" w256 {
                  frame 0, Default {
                    n172 = global write "Robot Global Data.vi" "Elevator Toggle"(u8 1 ("Elevator Toggle")) -> ()
                    n173 = call <vilib>:"WPI_MotorControlRefNum Registry Get.vi"("refnum name"="Elevator") -> ("MotorControlDevRef"=w259:T21)  [unwired: 9 in, 1 out]
                    n174 = call <vilib>:"WPI_MotorControlSetOutput.vi"("Output"=12.0 ("y"), "MotorControlDevRef"=w259) -> ()  [unwired: 8 in, 2 out]
                  }
                  frame 1 {
                    n175 = global write "Robot Global Data.vi" "Elevator Toggle"(u8 0 ("Elevator Toggle")) -> ()
                    n176 = call <vilib>:"WPI_MotorControlRefNum Registry Get.vi"("refnum name"="Elevator") -> ("MotorControlDevRef"=w262:T21)  [unwired: 9 in, 1 out]
                    n177 = call <vilib>:"WPI_MotorControlSetOutput.vi"("Output"=0.0 ("y"), "MotorControlDevRef"=w262) -> ()  [unwired: 8 in, 2 out]
                  }
                }
              }
              frame 1 {
              }
            }
          }
        }
      }
      frame #1 {
        n178 = call <vilib>:"WPI_JoystickRefNum Registry Get.vi"("refnum name"="Joystick 3") -> ("JoystickDevRef"=w268:T12)  [unwired: 9 in, 1 out]
        n179 = call <vilib>:"WPI_JoystickGet.vi"("JoystickDevRef"=w268) -> ("Buttons"=w269:T19)  [unwired: 4 in, 2 out]
        n180 = Unbundle By Name(w269) -> ("Button 4"=w266:bool)
        n181 = Boolean To (0,1)(Boolean=w266) -> (0, 1=w265:i16)
        n182 = global write "Robot Global Data.vi" "Elevator Button Prev"(w265) -> ()
      }
    }
    n183 = Wait (ms)(milliseconds to wait=u32 250) -> ()  [unwired: 1 out]
  }
  n184 = while {
    stop <- FALSE stop-if-true
    # "here's your data to use"
    # "make sure that\nv  is the same as what you sent"
    # "data has to be unflattened from string to be used"
    # "read UDP packet\nthis is the important part - you would normally open/close the socket elsewhere and read from it as needed\nyou can change the max size to reflect your packet, I'm going to leave it at the default (548)"
    # "open UDP connection\n - timeout defaults to 25000 ms\n - port can be changed as needed (see above comment for open field ports)"
    # "– UDP 1130: Dashboard-to-Robot control data, directional\n– UDP 1140: Robot-to-Dashboard status data, directional\n(2011 Team Update 5)"
    # "From Dashboard To Robot"
    n185 = Wait (ms)(milliseconds to wait=u32 200) -> ()  [unwired: 1 out]
    n186 = UDP Open(11:u16 1130 ("port")) -> (port=w280:refnum<k16>, 0:w279:errorcluster)  [unwired: 1 in, 4 out]
    n187 = UDP Read(connection ID=w280, 8:w279) -> (data out=w278:string, error out=w274:errorcluster, 3:w275:refnum<k16>)  [unwired: 4 out]
    n188 = UDP Close(connection ID=w275, 8:w274) -> ()  [unwired: 2 out]
    n189 = Unflatten From String(type=cluster{dbl, dbl} {0.0, 0.0}, binary string=w278) -> (value=w276:cluster{dbl, dbl})  [unwired: 1 in, 4 out]
    n190 = Unbundle(w276) -> (w271:dbl, w270:dbl)
    "Distance from dash" <- w271
    n191 = global write "Robot Global Data.vi" "Xerror"(w270) -> ()
    n192 = global write "Robot Global Data.vi" "Distance"(w271) -> ()
  }
  "Target Locked" <- w3
